vi "SubPanel Guest_Launch.vi"(0 "SubPanel":refnum<vi>, 9 "Timeout":i32=1000 format="%dmsec", 11 "error in":errorcluster) -> (4 "FTW Actor Connector":refnum<class "SubPanel Guest.lvclass">, 6 "Initialized Response":string, 8 "Instance Inbox Address":string, 15 "error out":errorcluster)   [LabVIEW 2013, in "SubPanel Guest.lvclass"]
uses:
  SubPanel Guest.lvclass
  Core/SubPanel Guest-Core_Process.vi
  source/actor/Connector/FTW-ActorConnector.lvclass
  templates/Actor Template/Core/Actor Template-Core.lvclass
  Core/SubPanel Guest-Core.lvclass
panel:
  in  "Boolean":bool
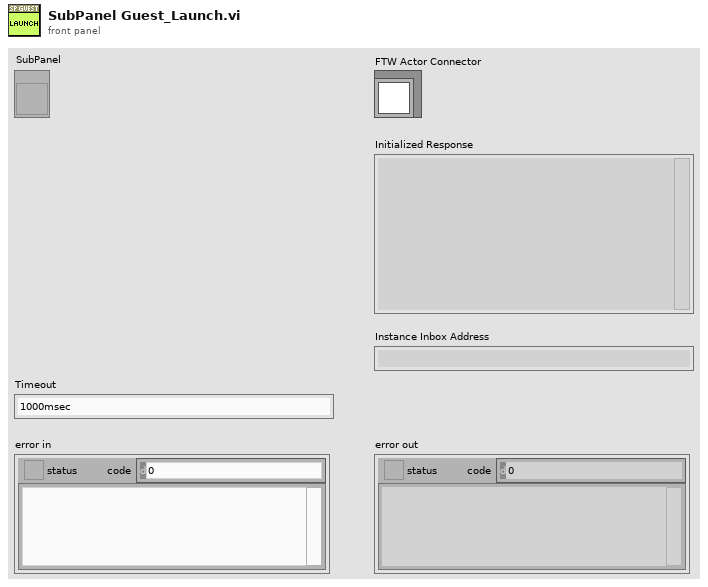
[diagram p1: front panel]
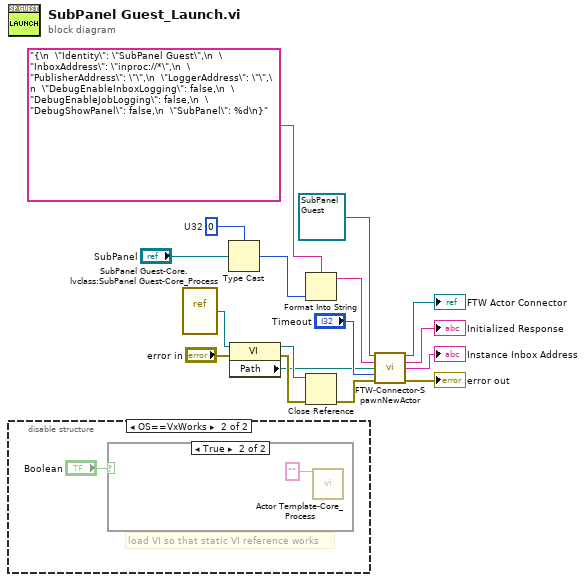
[diagram p0: block diagram]
diagram:
  w4 = u32 0  # U32
  n1 = disable-structure shown="OS==VxWorks" {
    frame condition #0 (active) {
    }
    frame condition #1 {
      # "load VI so that static VI reference works"
      n2 = case shown="True" "Boolean" {
        frame False {
        }
        frame True {
          n3 = call "Actor Template-Core_Process.vi"("FTW Actor Instance Configuration"="") -> ()  [unwired: 14 in, 1 out]
        }
      }
    }
  }
  n4 = vi-ref "SubPanel Guest-Core.lvclass:SubPanel Guest-Core_Process.vi"() -> (w11:refnum<vi>)
  n5 = Type Cast(type=w4, x="SubPanel") -> (*(type *) &x=w2:u32)
  n6 = property class="VI"(reference=w11, error in="error in") -> (reference out=w10:refnum<vi>, error out=w9:errorcluster, "Path"=w6:path)
  n7 = Format Into String(format string="{\n  \"Identity\": \"SubPanel Guest\",\n  \"InboxAddress\": \"inproc://*\",\n  \"PublisherAddress\": \"\",\n  \"LoggerAddress\": \"\",\n  \"DebugEnableInboxLogging\": false,\n  \"DebugEnableJobLogging\": false,\n  \"DebugShowPanel\": false,\n  \"SubPanel\": %d\n}" ("Configuration"), w2) -> (resulting string=w1:string)  [unwired: 2 in, 1 out]
  n8 = Close Reference(reference=w10, error in (no error)=w9) -> (error out=w7:errorcluster)
  n9 = call "FTW-Connector-SpawnNewActor.vi"("FTW Actor Connector Type"=refnum<class "SubPanel Guest.lvclass"> refnum ("TTK_Splashscreen.lvclass"), "Configuration"=w1, "Actor VI Filepath"=w6, "Timeout"="Timeout", "error in"=w7) -> ("FTW Actor Connector"=→"FTW Actor Connector":refnum<class "SubPanel Guest.lvclass">, "Initialized Response"=→"Initialized Response":string, "Instance Inbox Address"=→"Instance Inbox Address":string, "error out"=→"error out":errorcluster)  [unwired: 6 in, 1 out]
